vi "drive2.vi"() -> ()   [LabVIEW 2010, in "Test.lvrbt"]
uses:
  <vilib>/NXT/Subs/MotorOutput.ctl
  <vilib>/FTC/FTC Read Controller Packet.vi
  <vilib>/FTC/FTC Calculate Drive Power - Arcade Left.vi
  Test.lvrbt
panel:
  in  "Drive Power":i8=100 min=-100 max=100
  # "This VI was generated based on your configuration in the Remote Control Editor. You may modify the code as needed for your robot. To test this program for an FTC match, return to the Remote Control Editor, select the \"Run Program\" tab, and choose \"FTC Game\"."
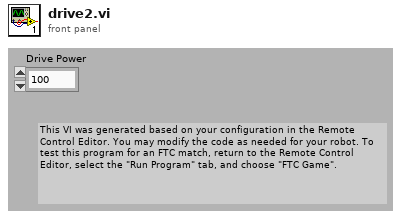
[diagram p1: front panel]
types:
  T1 = typedef "LVHSConnector.ctl" = cluster{"Hardware":string, "Flattened String":string}
  T2 = typedef "FTC ControllerState.ctl" = cluster{"Left X":i8, "Left Y":i8, "Right X":i8, "Right Y":i8, "Button Encoding 9-12":u8, "Button Encoding 1-8":u8, "POV":T3}
  T3 = typedef "FTC POVState.ctl" = i8
  T4 = typedef "MotorOutput.ctl" = u8
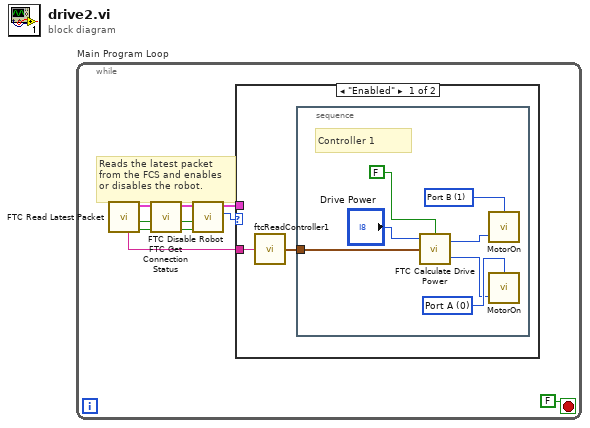
[diagram p0: block diagram]
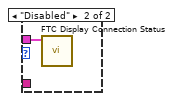
[diagram p2: hidden frame]
diagram:
  n1 = while "Main Program Loop" {
    stop <- FALSE stop-if-true
    # "Reads the latest packet\nfrom the FCS and enables\nor disables the robot."
    n2 = call <vilib>:"FTC Read Latest Packet.vi"() -> ("Packet Received?"=w8:bool, "Stopped?"=w5:bool, "NXT"=w7:T1, "Controller 1"=w9:string)  [unwired: 6 in, 2 out]
    n3 = call <vilib>:"FTC Get Connection Status.vi"("Packet Received?"=w8, "Stopped?"=w5, "NXT"=w7) -> ("Online?"=w2:bool, "Stopped?"=w3:bool, "NXT"=w4:T1)  [unwired: 5 in]
    n4 = call <vilib>:"FTC Disable Robot.vi"("Online?"=w2, "Stopped?"=w3, "NXT"=w4) -> ("Enabled?"=w6:enum16{"Disabled", "Enabled"}, "NXT"=w1:T1)  [unwired: 3 in]
    n5 = case "disableCase" shown="\"Enabled\"" w6 {
      tunnel: w9 -> [w12 _]
      tunnel: w1 -> [_ w20]
      frame "Enabled" {
        n6 = call "ftcReadController1"("Packet"=w12) -> ("Controller State"=w11:T2)  [unwired: 4 in]
        n7 = stacked-sequence "controller1Actions" {
          tunnel: w11 -> [w19]
          frame #0 {
            w14 = T4 0 items=["Port A"=0, "Port B"=1, "Port C"=2, "Ports A & B"=4, "Ports A & C"=5, "Ports B & C"=6, "All Ports"=3] ("Output Port (All Ports)")
            w16 = T4 1 items=["Port A"=0, "Port B"=1, "Port C"=2, "Ports A & B"=4, "Ports A & C"=5, "Ports B & C"=6, "All Ports"=3] ("Output Port (All Ports)")
            # "Controller 1"
            n8 = call-poly <vilib>:"FTC Calculate Drive Power.vi"("Reverse"=FALSE, "Controller State"=w19, "Power Level (50)"="Drive Power") -> ("Right Motor Power"=w13:i8, "Left Motor Power"=w15:i8)  [unwired: 1 in]
            n9 = call <vilib>:"MotorOn.vi"("Power (75)"=w15, "Output Port (All Ports)"=w16) -> ()  [unwired: 2 in, 1 out]
            n10 = call <vilib>:"MotorOn.vi"("Power (75)"=w13, "Output Port (All Ports)"=w14) -> ()  [unwired: 2 in, 1 out]
          }
        }
      }
      frame "Disabled" {
        n11 = call <vilib>:"FTC Display Connection Status.vi"("NXT"=w20) -> ()  [unwired: 10 in, 1 out]
      }
    }
  }
